vi "FXP2Int.vi"(9 "Output Bit resolution":i8=12, 10 "Multiplier":fxp<+,18,-1>=0.39999961853027344, 11 "Input (FXP)":fxp<+/-,18,5>) -> (3 "Output (Int)":i16)   [LabVIEW 2019, in "FPGA functions.lvlib"]
doc: "Converts Fixed-Point (±16,4) into integer of the requested number of bits.\n\nCheck scaling to match the range and resolution of DAC hardware"
uses:
  FPGA functions.lvlib
  <vilib>/Platform/TimedLoop/XDataNode/timing_clust.ctl
  <vilib>/Platform/TimedLoop/XDataNode/nitl_modes.ctl
  <vilib>/Platform/TimedLoop/XDataNode/wakeup.ctl
  <vilib>/Platform/TimedLoop/XDataNode/XDataNode.xnode
  <vilib>/rvi/FXPMathLib/FxpMul/XNode/nifxpmath_Multiplier.xnode
  <vilib>/Platform/TimedLoop/XDataNode/XDNodeRunTimeDep.lvlib
  <vilib>/rvi/FXPMathLib/sim/FxpSim.dll
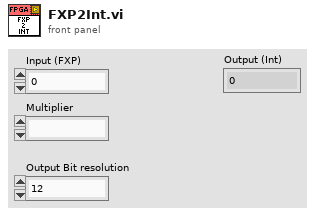
[diagram p1: front panel]
types:
  T1 = typedef "XDNodeRunTimeDep.lvlib/timing_clust.ctl" = cluster{"Expected End [f-1]":u64, "Actual End [f-1]":u64, "Finished Late? [f-1]":bool, "Expected End [i-1]":u64, "Actual End [i-1]":u64, "Finished Late? [i-1]":bool, "Expected Start [i]":u64, "Actual Start [i]":u64, "Expected Start [f]":u64, "Actual Start [f]":u64, "Source Name":string, "Structure Name":string, "Period":i64, "Deadline":i64, "Offset":i64, "Start":i64, "Priority":i32, "Timeout":i32, "Mode":T2, "Wakeup Reason":T3, "Error":errorcluster, "Source Type":string, "Secondary Source Type":string, "Global End Time":u64, "Global Start Time":u64, "Frame Duration":u64, "Iteration Duration":u64, "Assigned CPU":i32, "I/O Scan Engine Mode":u32}
  T2 = typedef "XDNodeRunTimeDep.lvlib/nitl_modes.ctl" = enum32{"No Change", "Process missed periods, maintain original phase", "Discard missed periods, maintain original phase", "Process missed periods, ignore original phase", "Discard missed periods, ignore original phase"}
  T3 = typedef "XDNodeRunTimeDep.lvlib/wakeup.ctl" = enum32{"Normal", "Aborted", "Asynchronous wakeup", "Timing source error", "Timed loop error", "Timeout"}
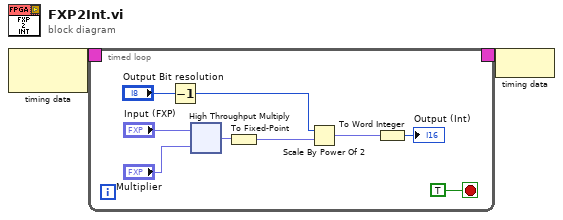
[diagram p0: block diagram]
diagram:
  n1 = node-c288() -> (w2:T1)  [unwired: 1 in]
  n2 = timed-loop {
    timing: w2 -> [_]
    timing-out: [_] -> w1
    stop <- TRUE stop-if-true
    n3 = Decrement(x="Output Bit resolution") -> (x-1=w7:i8)
    n4 = xnode ("High Throughput Multiply")("x"="Input (FXP)", "y"="Multiplier") -> ("x*y"=w4:fxp<+/-,18,1>)
    n5 = To Fixed-Point(number=w4) -> (fixed-point=w11:fxp<+/-,32,13>)  [unwired: 1 in]
    n6 = Scale By Power Of 2(n=w7, x=w11) -> (x*2^n=w3:fxp<+/-,32,13>)
    n7 = To Word Integer(number=w3) -> (16bit integer=→"Output (Int)":i16)
  }
  n8 = node-c288(w1) -> ()
